vi "Is JSON Parseable.vi"(8 "error in":errorcluster, 11 "<JSON>":string) -> (0 "error out":errorcluster, 2 "Is Valid?":bool, 3 "Pretty <JSON>":string)   [LabVIEW 2023, in "Configuration UI Actor.lvlib" / "Configuration UI Actor.lvclass"]
uses:
  Configuration UI Actor.lvclass
  Configuration UI Actor.lvclass/Configuration UI Actor.ctl
  <vilib>/JDP Science/JSONtext/JSONtext.lvlib
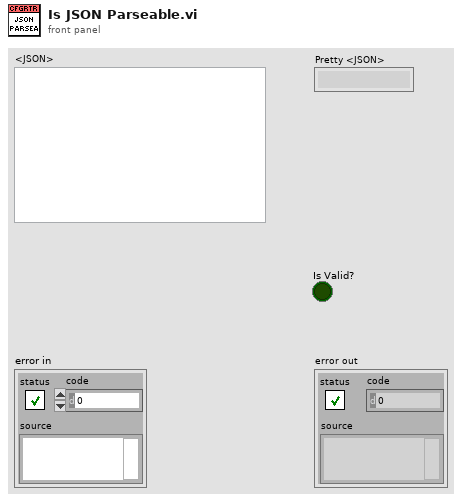
[diagram p1: front panel]
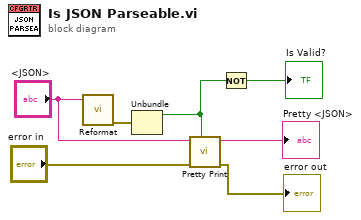
[diagram p0: block diagram]
diagram:
  n1 = call <vilib>:"Reformat.vi"("JSON"="<JSON>") -> ("error out"=w3:errorcluster)  [unwired: 7 in, 3 out]
  n2 = Unbundle(w3) -> ("status"=w2:bool)  [unwired: 2 out]
  n3 = call <vilib>:"Pretty Print.vi"("Comment out unparsable lines"=w2, "error in (no error)"="error in", "JSON"="<JSON>") -> ("error out"=→"error out":errorcluster, "<JSON>"=→"Pretty <JSON>":string)  [unwired: 6 in, 1 out]
  n4 = Not(x=w2) -> (.not. x?=→"Is Valid?":bool)
